vi "Windows - Display Turbine Status.vi"() -> ()   [LabVIEW 2012]
uses:
  Type Defs/Command Datatype.ctl
panel:
  in  "Turbine PWM Period (mS)":dbl
  in  "Turbine PWM Duty Cycle (%)":dbl min=0.0 max=100.0 step=1.0
  in  "Trigger Acq":bool
  out "FFT":dbl[](graph)
  out "Accelerometer":dbl[](graph)
  out "Tach Velocity (RPM)":dbl(knob) scale=0.0..6000.0
  in  "stop":bool
  out "Temperature":dbl(graph)
  # "Turbine Test"
  # "Turbine Speed Control"
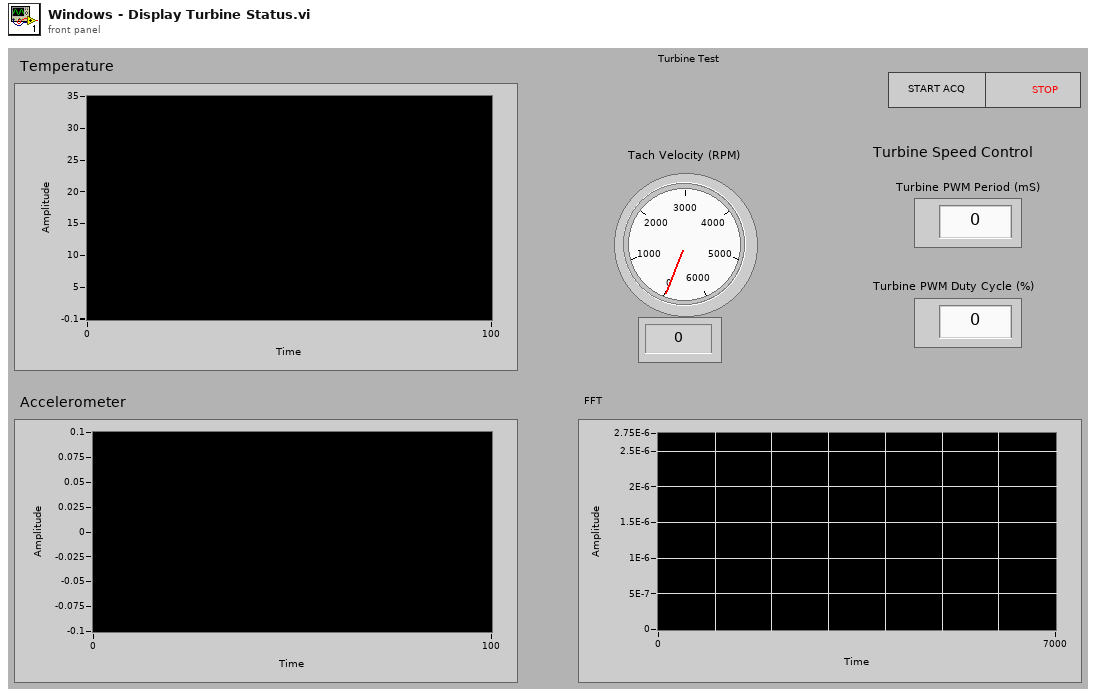
[diagram p1: front panel]
types:
  T1 = typedef "Command Datatype.ctl" = cluster{"Cmd":string, "Data":variant}
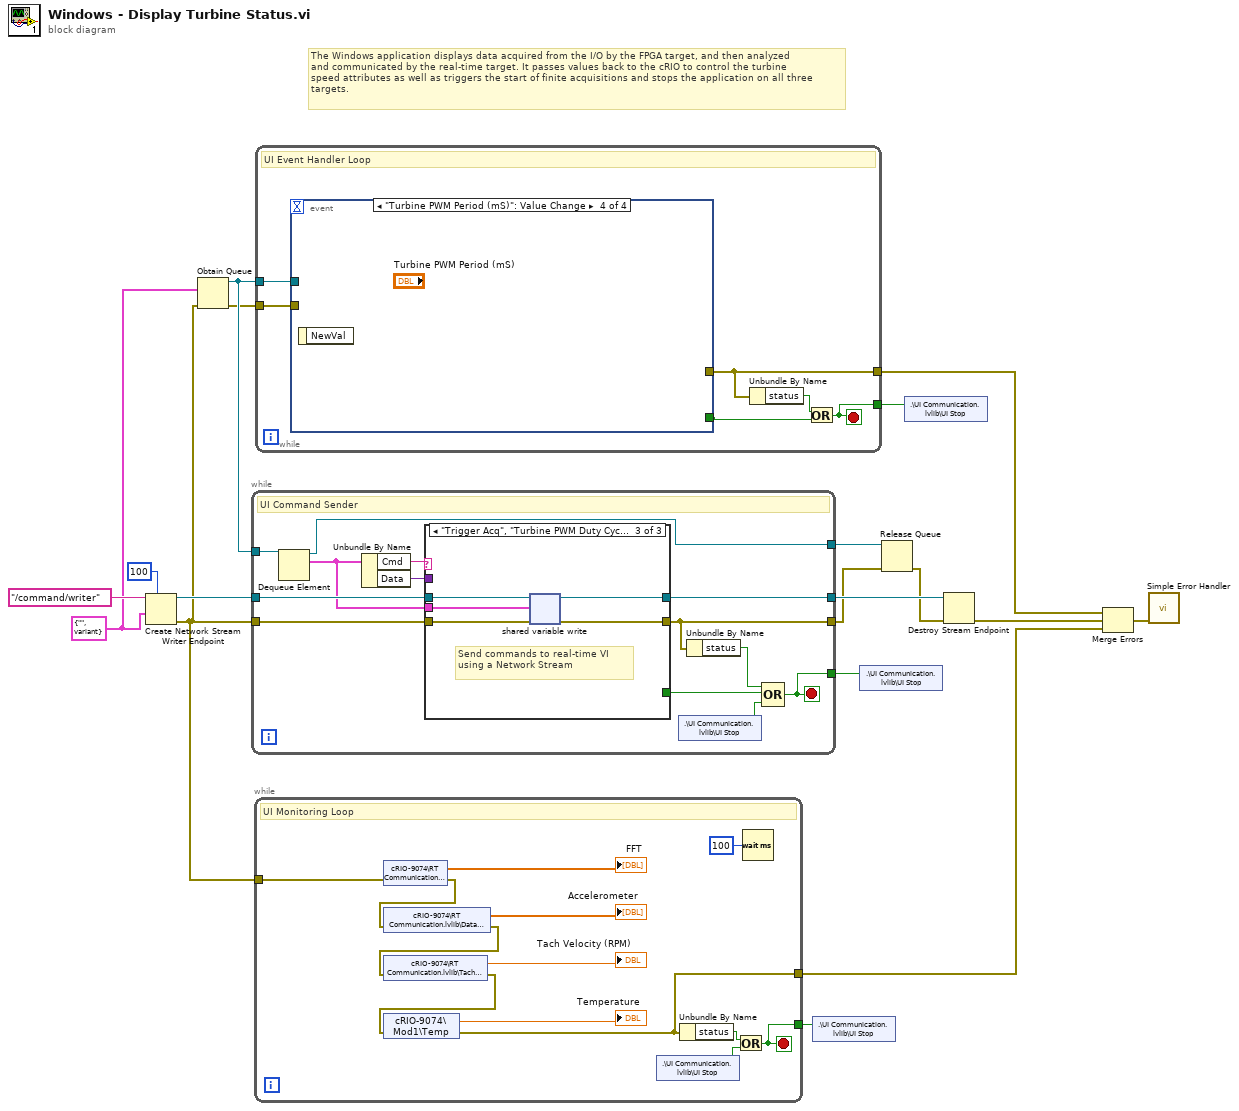
[diagram p0: block diagram]
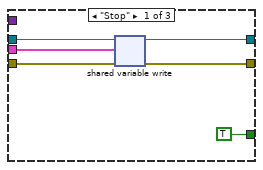
[diagram p2: hidden frame]
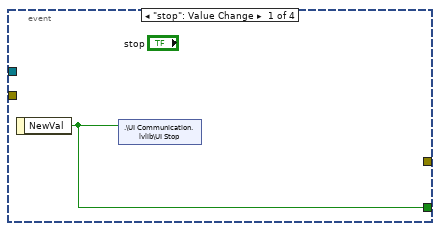
[diagram p4: hidden frame]
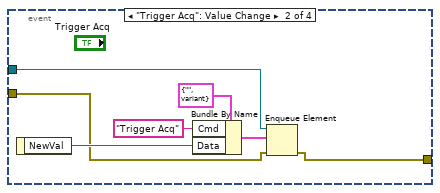
[diagram p5: hidden frame]
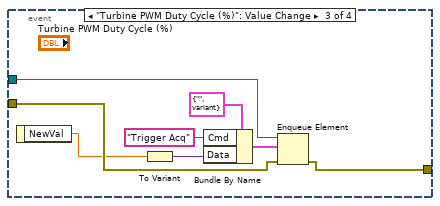
[diagram p6: hidden frame]
diagram:
  w15 = T1 {"Cmd"="", "Data"=variant} ("Cluster")
  # "The Windows application displays data acquired from the I/O by the FPGA target, and then analyzed\nand communicated by the real-time target. It passes values back to the cRIO to control the turbine\nspeed attributes as well as triggers the start of finite acquisitions and stops the application on all three\ntargets."
  n1 = Create Network Stream Writer Endpoint(7:100 ("writer buffer size"), 9:w15, 11:"/command/writer" ("writer name")) -> (0:w11:errorcluster, 3:w18:refnum<k21>)  [unwired: 4 in]
  n2 = Obtain Queue(element data type=w15, error in (no error)=w11) -> (queue out=w14:refnum<queue>, error out=w13:errorcluster)  [unwired: 3 in, 1 out]
  n3 = while {
    tunnel: w18 -> [w30]
    tunnel: w14 -> [w31]
    tunnel: w11 -> [w29]
    tunnel: [w26] -> w6
    tunnel: [w25] -> w12
    tunnel: [w20] -> w9
    tunnel: [w19] -> w7
    stop <- w20 stop-if-true
    # "UI Command Sender"
    n4 = Dequeue Element(queue=w31) -> (queue out=w19:refnum<queue>, element=w27:T1)  [unwired: 2 in, 2 out]
    n5 = Unbundle By Name(w27) -> ("Cmd"=w28:string, "Data"=w24:variant)
    n6 = case shown="\"Trigger Acq\", \"Turbine PWM Duty Cycle\", \"Turbine PWM Period\"" w28 {
      tunnel: w30 -> [w33 w39 w44]
      tunnel: w29 -> [w36 w38 w43]
      tunnel: [w35 w38 w42] -> w26
      tunnel: w27 -> [w34 _ w41]
      tunnel: [TRUE _ _] -> w22
      tunnel: [w32 w39 w40] -> w25
      tunnel: w24 -> [_ _ _]
      frame "Stop" {
        n7 = shared-variable-write(w33, w36, w34) -> (w32:refnum<k21>, w35:errorcluster)  [unwired: 1 in, 1 out]
      }
      frame Default {
      }
      frame "Trigger Acq", "Turbine PWM Duty Cycle", "Turbine PWM Period" {
        # "Send commands to real-time VI using a Network Stream"
        n8 = shared-variable-write(w44, w43, w41) -> (w40:refnum<k21>, w42:errorcluster)  [unwired: 1 in, 1 out]
      }
    }
    n9 = shared-variable ".\\UI Communication.lvlib\\UI Stop"() -> (w21:bool)  [unwired: 1 in, 1 out]
    n10 = Unbundle By Name(w26) -> ("status"=w23:bool)
    n11 = Compound Arithmetic op=OR(w23, w22, w21) -> (w20:bool)
  }
  n12 = while {
    tunnel: w11 -> [w52]
    tunnel: [w46] -> w8
    tunnel: [w45] -> w2
    stop <- w46 stop-if-true
    # "UI Monitoring Loop"
    n13 = shared-variable "cRIO-9074\\RT Communication.lvlib\\FFT"(error in=w52) -> (→"FFT":dbl[], error out=w51:errorcluster)
    n14 = shared-variable "cRIO-9074\\RT Communication.lvlib\\Data Subset"(error in=w51) -> (→"Accelerometer":dbl[], error out=w50:errorcluster)
    n15 = shared-variable "cRIO-9074\\RT Communication.lvlib\\Tach RPMs"(error in=w50) -> (→"Tach Velocity (RPM)":dbl, error out=w49:errorcluster)
    n16 = shared-variable "cRIO-9074\\Mod1\\Temp"(error in=w49) -> (→"Temperature":dbl, error out=w45:errorcluster)
    n17 = shared-variable ".\\UI Communication.lvlib\\UI Stop"() -> (w48:bool)  [unwired: 1 in, 1 out]
    n18 = Unbundle By Name(w45) -> ("status"=w47:bool)
    n19 = Or(x=w47, y=w48) -> (x .or. y?=w46:bool)
    n20 = Wait (ms)(milliseconds to wait=u32 100) -> ()  [unwired: 1 out]
  }
  n21 = while {
    tunnel: w14 -> [w63]
    tunnel: w13 -> [w62]
    tunnel: [w60] -> w4
    tunnel: [w58] -> w10
    stop <- w58 stop-if-true
    # "UI Event Handler Loop"
    n22 = event shown="[3] \"Turbine PWM Period (mS)\": Value Change" {
      selector: _ -> [_ _ _ _]
      dyn-events: _ -> [_ _ _ _]
      timeout: _ -> [_ _ _ _]
      tunnel: w63 -> [_ w68 w76 _]
      tunnel: w62 -> [_ w66 w75 _]
      tunnel: [_ w65 w74 _] -> w60
      tunnel: [w64 _ _ _] -> w59
      event "stop": Value Change {
        n23 = event-data() -> ("NewVal"=w64:bool)  [unwired: 1 in]
        n24 = shared-variable ".\\UI Communication.lvlib\\UI Stop"(w64) -> ()  [unwired: 1 in, 1 out]
      }
      event "Trigger Acq": Value Change {
        n25 = event-data() -> ("NewVal"=w69:bool)  [unwired: 1 in]
        n26 = Bundle By Name(cluster=T1 {"Cmd"="", "Data"=variant} ("Cluster"), "Cmd"="Trigger Acq", "Data"=w69) -> (w67:T1)
        n27 = Enqueue Element(queue=w68, element=w67, error in (no error)=w66) -> (error out=w65:errorcluster)  [unwired: 1 in, 2 out]
      }
      event "Turbine PWM Duty Cycle (%)": Value Change {
        n28 = event-data() -> ("NewVal"=w73:dbl)  [unwired: 1 in]
        n29 = To Variant(anything=w73) -> (Variant=w72:variant)
        n30 = Bundle By Name(cluster=T1 {"Cmd"="", "Data"=variant} ("Cluster"), "Cmd"="Trigger Acq", "Data"=w72) -> (w77:T1)
        n31 = Enqueue Element(queue=w76, element=w77, error in (no error)=w75) -> (error out=w74:errorcluster)  [unwired: 1 in, 2 out]
      }
      event "Turbine PWM Period (mS)": Value Change {
        n32 = event-data() -> ()  [unwired: 1 in, 1 out]
      }
    }
    n33 = Unbundle By Name(w60) -> ("status"=w61:bool)
    n34 = Or(x=w61, y=w59) -> (x .or. y?=w58:bool)
  }
  n35 = shared-variable ".\\UI Communication.lvlib\\UI Stop"(w8) -> ()  [unwired: 1 in, 1 out]
  n36 = shared-variable ".\\UI Communication.lvlib\\UI Stop"(w9) -> ()  [unwired: 1 in, 1 out]
  n37 = Release Queue(queue=w7, error in (no error)=w6) -> (error out=w5:errorcluster)  [unwired: 1 in, 2 out]
  n38 = shared-variable ".\\UI Communication.lvlib\\UI Stop"(w10) -> ()  [unwired: 1 in, 1 out]
  n39 = Destroy Stream Endpoint(8:w5, 11:w12) -> (0:w3:errorcluster)
  n40 = Merge Errors(w4, w3, w2) -> (w1:errorcluster)
  n41 = call <vilib>:"Simple Error Handler.vi"("error in (no error)"=w1) -> ()  [unwired: 4 in, 5 out]
